vi "disable section in init.vi"(10 "Boolean":bool, 11 "GObject in":refnum<vi>) -> (0 "error out":errorcluster)   [LabVIEW 2013, in "FixedChannelTBModuleDecideFeatures.lvclass"]
uses:
  FixedChannelTBModuleDecideFeatures.lvclass
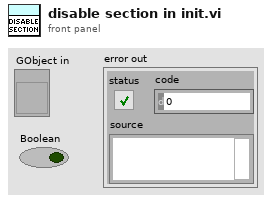
[diagram p1: front panel]
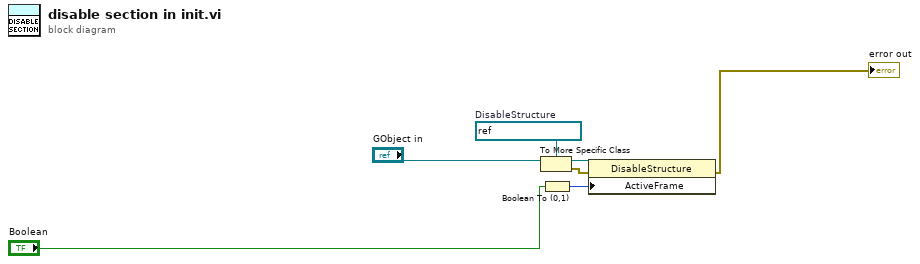
[diagram p0: block diagram]
diagram:
  w2 = refnum<vi> refnum  # DisableStructure
  n1 = To More Specific Class(target class=w2, reference="GObject in") -> (specific class reference=w1:refnum<vi>, error out=w6:errorcluster)  [unwired: 1 in]
  n2 = Boolean To (0,1)(Boolean="Boolean") -> (0, 1=w4:i16)
  n3 = property class="DisableStructure"(reference=w1, error in=w6, "ActiveFrame"=w4) -> (error out=→"error out":errorcluster)  [unwired: 1 out]
